vi "2.0.-Lectura de Imagen.vi"() -> ()   [LabVIEW 2020]
panel:
  out "new picture":picture
  in  "File Path":path
  out "Image":T1(plugin-control)
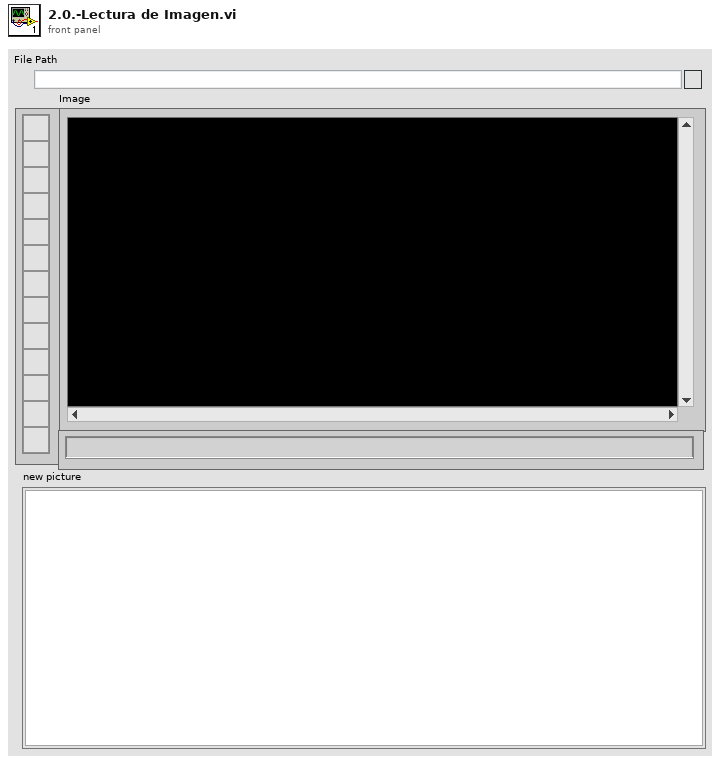
[diagram p1: front panel]
types:
  T1 = typedef "IMAQ Image.ctl" = refnum<image>
  T2 = typedef "Image Type" = u32
  T3 = typedef "imagedata.ctl" = cluster{"image type":i32, "image depth":i32, "image":u8[], "mask":u8[], "colors":u32[], "Rectangle":cluster{"left":i16, "top":i16, "right":i16, "bottom":i16}}
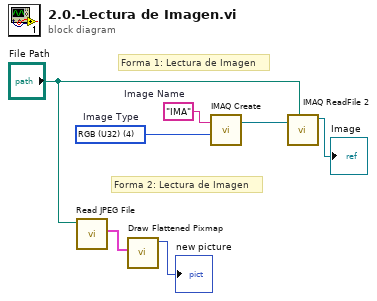
[diagram p0: block diagram]
diagram:
  w4 = "IMA"  # Image Name
  w5 = T2 4 items=["Grayscale (U8)", "Grayscale (I16)", "Grayscale (SGL)", "Complex (CSG)", "RGB (U32)", "HSL (U32)", "RGB (U64)", "Grayscale (U16)"]  # Image Type
  # "Forma 2: Lectura de Imagen"
  # "Forma 1: Lectura de Imagen"
  n1 = call <vilib>:"Read JPEG File.vi"("path to JPEG file"="File Path") -> ("image data"=w2:T3)  [unwired: 8 in, 2 out]
  n2 = call <vilib>:"Draw Flattened Pixmap.vi"("image data"=w2) -> ("new picture"=→"new picture":picture)  [unwired: 8 in]
  n3 = call "IMAQ Create"("Image Name"=w4, "Image Type"=w5) -> ("New Image"=w6:T1)  [unwired: 3 in, 1 out]
  n4 = call "IMAQ ReadFile 2"("File Path"="File Path", "Image"=w6) -> ("Image Out"=→"Image":T1)  [unwired: 5 in, 4 out]
